vi "GetOneFrameTimeout.vi"(0 "handle":u64, 5 "pData":u8[](array[numeric]), 7 "nDataSize":u32, 9 "nMsec":u32, 11 "error in (no error)":errorcluster caption="错误输入（无错误）") -> (4 "handle out":u64, 6 "function return":i32, 8 "pData Out":u8[](array[numeric]), 10 "pFrameInfoEx out":T1, 15 "error out":errorcluster caption="错误输出")   [LabVIEW 2011, in "MvCameraControl.lvlib"]
uses:
  MvCameraControl.lvlib
  MvCameraControl.dll
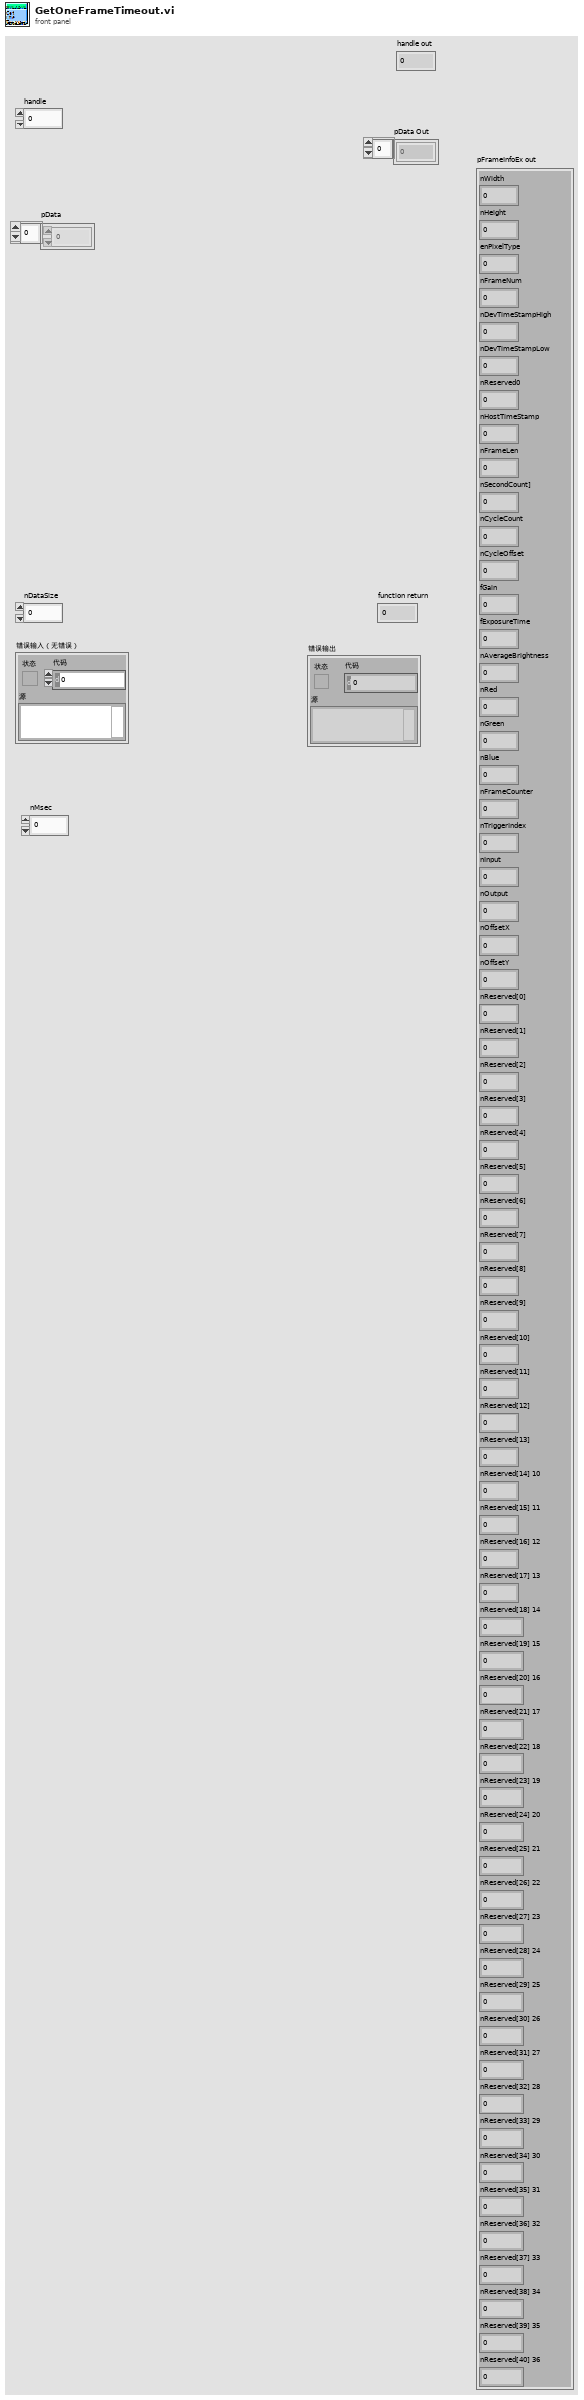
[diagram p1: front panel]
types:
  T1 = cluster{"nWidth":u16, "nHeight":u16, "enPixelType":i32, "nFrameNum":u32, "nDevTimeStampHigh":u32, "nDevTimeStampLow":u32, "nReserved0":u32, "nHostTimeStamp":i64, "nFrameLen":u32, "nSecondCount]":u32, "nCycleCount":u32, "nCycleOffset":u32, "fGain":u32, "fExposureTime":u32, "nAverageBrightness":u32, "nRed":u32, "nGreen":u32, "nBlue":u32, "nFrameCounter":u32, "nTriggerIndex":u32, "nInput":u32, "nOutput":u32, "nOffsetX":u32, "nOffsetY":u32, "nReserved[0]":u32, "nReserved[1]":u32, "nReserved[2]":u32, "nReserved[3]":u32, "nReserved[4]":u32, "nReserved[5]":u32, "nReserved[6]":u32, "nReserved[7]":u32, "nReserved[8]":u32, "nReserved[9]":u32, "nReserved[10]":u32, "nReserved[11]":u32, "nReserved[12]":u32, "nReserved[13]":u32, "nReserved[14] 10":u32, "nReserved[15] 11":u32, "nReserved[16] 12":u32, "nReserved[17] 13":u32, "nReserved[18] 14":u32, "nReserved[19] 15":u32, "nReserved[20] 16":u32, "nReserved[21] 17":u32, "nReserved[22] 18":u32, "nReserved[23] 19":u32, "nReserved[24] 20":u32, "nReserved[25] 21":u32, "nReserved[26] 22":u32, "nReserved[27] 23":u32, "nReserved[28] 24":u32, "nReserved[29] 25":u32, "nReserved[30] 26":u32, "nReserved[31] 27":u32, "nReserved[32] 28":u32, "nReserved[33] 29":u32, "nReserved[34] 30":u32, "nReserved[35] 31":u32, "nReserved[36] 32":u32, "nReserved[37] 33":u32, "nReserved[38] 34":u32, "nReserved[39] 35":u32, "nReserved[40] 36":u32}
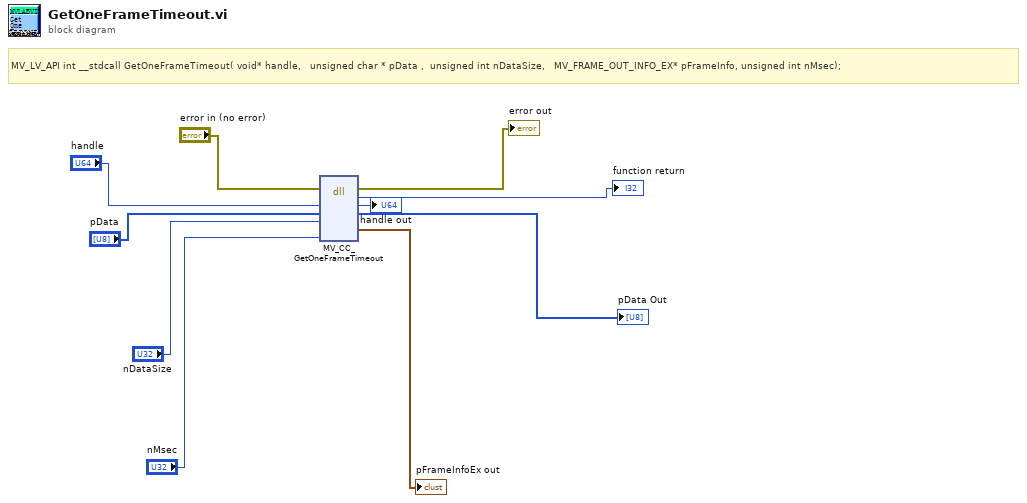
[diagram p0: block diagram]
diagram:
  # "MV_LV_API int __stdcall GetOneFrameTimeout( void* handle,   unsigned char * pData ,  unsigned int nDataSize,   MV_FRAME_OUT_INFO_EX* pFrameInfo, unsigned int nMsec);"
  n1 = dll-call lib="MvCameraControl.dll" fn="MV_CC_GetOneFrameTimeout"(error in="error in (no error)", "handle"="handle", "pData"="pData", "nDataSize"="nDataSize", "nMsec"="nMsec") -> (error out=→"error out":errorcluster, "返回类型"=→"function return":i32, "handle"=→"handle out":u64, "pData"=→"pData Out":u8[], "pFrameInfoEx out"=→"pFrameInfoEx out":T1)  [unwired: 5 in, 1 out]
